vi "DXD Pressure Sensors Control.vi"(9 "Record Pressure?":bool, 10 "Unit":T3(ring), 11 "VISA Refnum in":refnum<visa-resource-name>="COM6") -> (1 "Cluster 2":T2, 2 "Cluster":T1, 3 "Cluster 3":T1)   [LabVIEW 2015]
uses:
  CFR LabVIEW Software/DoE_Control - JMW 03032016/DoE_Control_v5 Folder/LabView VI Drivers for Heise DXD Digital Pressure Transducer/Type Defs/DXD Address.ctl
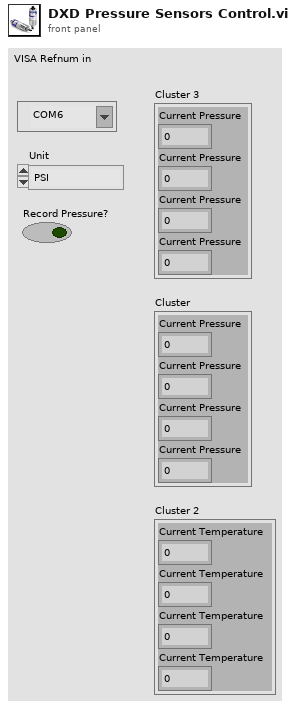
[diagram p1: front panel]
types:
  T1 = cluster{"Current Pressure":dbl, "Current Pressure":dbl, "Current Pressure":dbl, "Current Pressure":dbl}
  T2 = cluster{"Current Temperature":dbl, "Current Temperature":dbl, "Current Temperature":dbl, "Current Temperature":dbl}
  T3 = enum16{"PSI", "Bar", "cm H2O", "ft H2O", "hectoPascal", "in Hg", "in H2O", "kiloPascal", "milliBar", "mmHg", "MegaPascal", "Numeric Pressure"}
  T4 = typedef "DXD Address.ctl" = i32
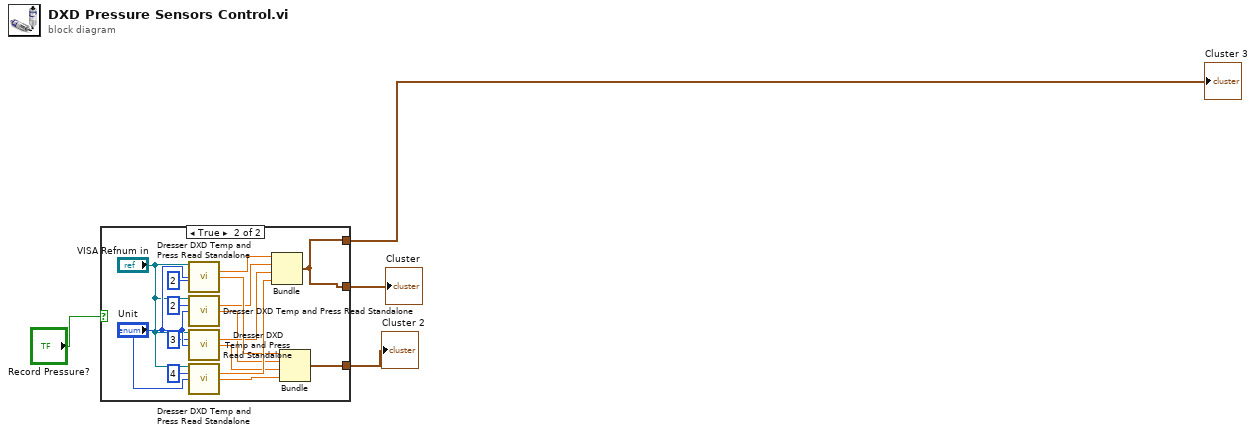
[diagram p0: block diagram]
diagram:
  n1 = case shown="True" "Record Pressure?" {
    tunnel: [_ w5] -> w1
    tunnel: [_ w6] -> w3
    tunnel: [_ w5] -> w4
    frame False {
    }
    frame True {
      n2 = call "Dresser DXD Temp and Press Read Standalone.vi"("Serial Port (COM1)"="VISA Refnum in", "DXD Address (1)"=T4 2, "Pressure Units (PSI)"="Unit") -> ("Current Pressure"=w10:dbl, "Current Temperature"=w13:dbl)  [unwired: 9 in, 2 out]
      n3 = call "Dresser DXD Temp and Press Read Standalone.vi"("Serial Port (COM1)"="VISA Refnum in", "DXD Address (1)"=T4 2, "Pressure Units (PSI)"="Unit") -> ("Current Pressure"=w11:dbl, "Current Temperature"=w9:dbl)  [unwired: 9 in, 2 out]
      n4 = call "Dresser DXD Temp and Press Read Standalone.vi"("Serial Port (COM1)"="VISA Refnum in", "DXD Address (1)"=T4 3, "Pressure Units (PSI)"="Unit") -> ("Current Pressure"=w12:dbl, "Current Temperature"=w8:dbl)  [unwired: 9 in, 2 out]
      n5 = call "Dresser DXD Temp and Press Read Standalone.vi"("Serial Port (COM1)"="VISA Refnum in", "DXD Address (1)"=T4 4, "Pressure Units (PSI)"="Unit") -> ("Current Pressure"=w14:dbl, "Current Temperature"=w7:dbl)  [unwired: 9 in, 2 out]
      n6 = Bundle("Current Pressure"=w10, "Current Pressure"=w11, "Current Pressure"=w12, "Current Pressure"=w14) -> (w5:T1)  [unwired: 1 in]
      n7 = Bundle("Current Temperature"=w13, "Current Temperature"=w9, "Current Temperature"=w8, "Current Temperature"=w7) -> (w6:T2)  [unwired: 1 in]
    }
  }
  "Cluster" <- w4
  "Cluster 2" <- w3
  "Cluster 3" <- w1
